vi "Generate Data.vi"(8 "Error In":errorcluster, 11 "String Data In":refnum<class "String Data.lvclass">) -> (0 "Error Out":errorcluster, 3 "String Data Out":refnum<class "String Data.lvclass">)   [LabVIEW 2022 SP3, in "String Data.lvclass"]
doc: "This VI generates a string data."
uses:
  String Data.lvclass
panel:
  out "String Data":string
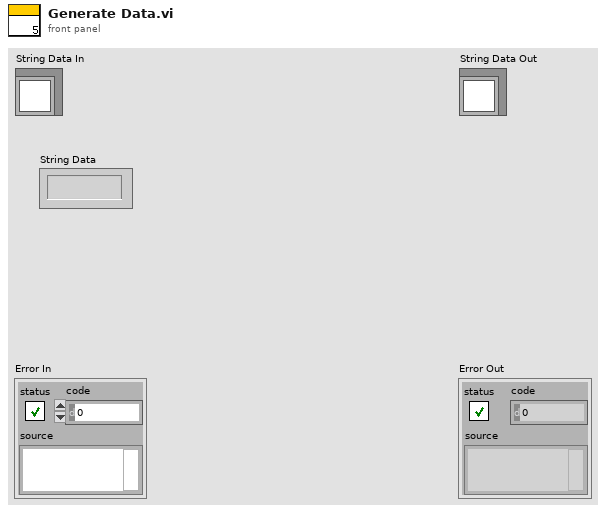
[diagram p1: front panel]
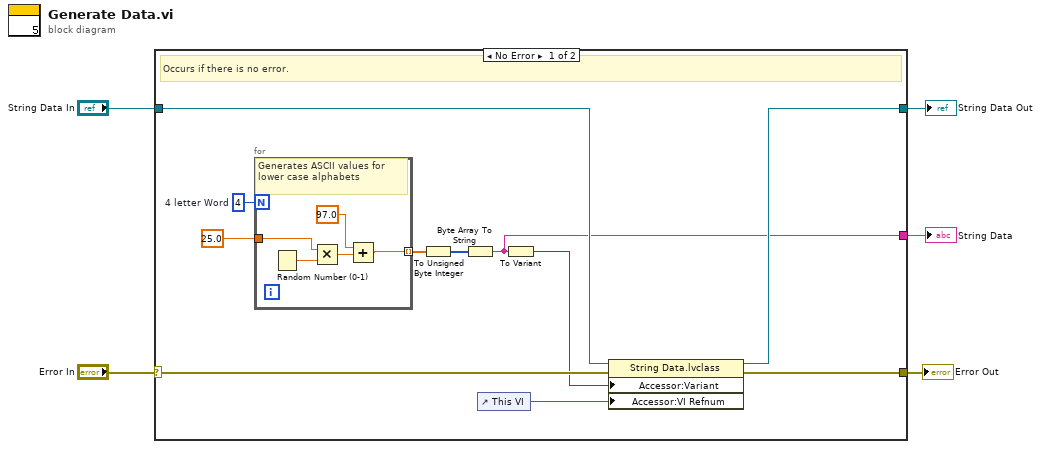
[diagram p0: block diagram]
diagram:
  n1 = case shown="No Error" "Error In" {
    selector: "Error In" -> [w16 w23]
    tunnel: [w9 w23] -> w4
    tunnel: [w8 w22] -> w2
    tunnel: "String Data In" -> [w11 w22]
    tunnel: [w6 _] -> w1
    frame No Error {
      w15 = 4  # 4 letter Word
      # "Occurs if there is no error."
      n2 = for {
        N: w15 -> [_]
        tunnel: 25.0 -> [w20]
        tunnel: [w17] -> w13 mode=indexing
        # "Generates ASCII values for lower case alphabets"
        n3 = Random Number (0-1)() -> (number: 0 to 1=w21:dbl)
        n4 = Multiply(x=w20, y=w21) -> (x*y=w19:dbl)
        n5 = Add(x=97.0, y=w19) -> (x+y=w17:dbl)
      }
      n6 = To Unsigned Byte Integer(number=w13) -> (unsigned 8bit integer=w12:u8[])
      n7 = Byte Array To String(unsigned byte array=w12) -> (string=w6:string)
      n8 = control-ref of="This VI"() -> (w7:refnum<vi>)
      n9 = To Variant(anything=w6) -> (Variant=w10:variant)
      n10 = property class="String Data.lvclass"(reference=w11, error in=w16, "Accessor:Variant"=w10, "Accessor:VI Refnum"=w7) -> (reference out=w8:refnum<class "String Data.lvclass">, error out=w9:errorcluster)
    }
    frame Error {
      # "Occurs if there is any error."
    }
  }
  "Error Out" <- w4
  "String Data Out" <- w2
  "String Data" <- w1
